vi "PosStrikerAnguloAttackerV2.vi"(9 "atacando contra":bool, 10 "IA State":T1={"our_robots"=[], "enemy_robots"=[], "balls"=[], "geometry"={"line_width"=0, "field_length"=0, "field_width"=0, "boundary_width"=0, "referee_width"=0, "goal_width"=0, "goal_depth"=0, "goal_wall_width"=0, "center_circle_radius"=0, "defense_radius"=0, "defense_stretch"=0, "free_kick_from_defense_dist"=0, "penalty_spot_from_field_line_dist"=0, "penalty_line_from_spot_dist"=0}, "IA Judge"={"stage"="", "command"="", "our_goalie_id"=0.0, "enemy_goalie_id"=0.0, "command enum"=enum."Halt", "Time"=enum."Azul"}, "Received Timestamp"=timestamp(0 s since 1904-01-01), "Events"={"Touch"=FALSE, "Ball out"=FALSE, "id touch"=0.0, "Ball out of \nVision"=FALSE, "Ball inside \nGoalie area"=FALSE, "Robot not responding"=FALSE, "Robots responding status"=[1.0, 1.0, 1.0, 1.0, 1.0, 1.0], "Enemy Ball \nPossession"=FALSE, "Pass State"=FALSE, "id end of pass"=0.0, "Kick"=FALSE, "Id ini Possession"=0.0, "Ball Possesion"=FALSE, "Id Possesion"=0.0, "Direct Kick"=FALSE}}) -> (0 "YdoAttacker 2":dbl, 1 "AttackerPositive?":bool, 2 "theta final":dbl, 3 "XdoAttacker 2":dbl)   [LabVIEW 2017]
uses:
  Core/AI Input.ctl
  Core/AI Robot.ctl
  Intel/Functions Enum.ctl
  Intel/AttackerStates.ctl
  Path Planning/RRT/PathDests.ctl
  Path Planning/RRT/PathDest.ctl
  Core/AI Ball.ctl
  Core/Field Size.ctl
  Core/AI Judge.ctl
  Intel/Command Enum.ctl
  Events/Events.ctl
panel:
  in  "valor de theta 3":dbl
  in  "tamanho do intervalo 3":dbl
  in  "inicio do intervalo 3":dbl
  in  "fim do intervalo 3":dbl
  in  "Contador 4":dbl
  in  "Array 3":dbl[](array[numeric])=[0.0, 0.0, 0.0, 0.0, 0.0, 0.0]
  in  "valor de theta 2":dbl
  in  "tamanho do intervalo 2":dbl
  in  "inicio do intervalo 2":dbl
  in  "fim do intervalo 2":dbl
  in  "Contador 3":dbl
  in  "Array 2":dbl[](array[numeric])=[0.0, 0.0, 0.0, 0.0, 0.0, 0.0]
  in  "XdoAttacker":dbl
  in  "YdoAttacker":dbl
  in  "RobôsParaAnalisar":dbl[][](array[numeric])=[[99999.0, 99999.0], [99999.0, 99999.0], [99999.0, 99999.0], [99999.0, 99999.0], [99999.0, 99999.0], [99999.0, 99999.0], [99999.0, 99999.0]]
  in  "Contador":dbl
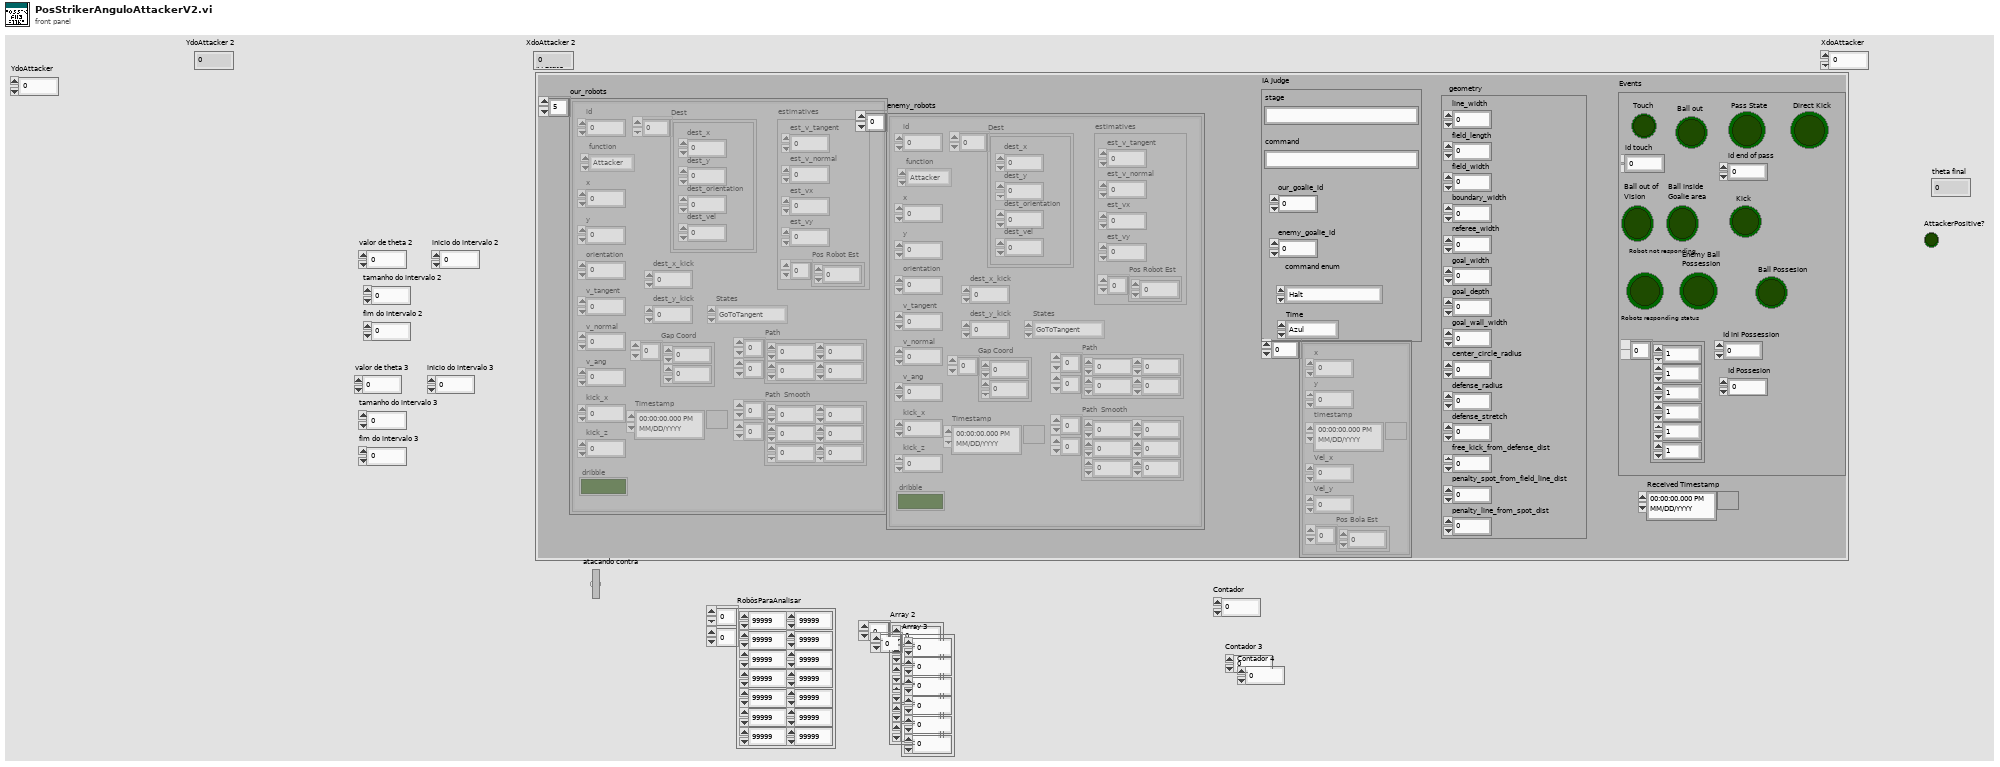
[diagram p1: front panel]
types:
  T1 = typedef "AI Input.ctl" = cluster{"our_robots":T2[], "enemy_robots":T2[], "balls":T7[], "geometry":T8, "IA Judge":T9, "Received Timestamp":timestamp, "Events":T11}
  T2 = typedef "AI Robot.ctl" = cluster{"id":u32, "function":T3, "x":dbl, "y":dbl, "orientation":dbl, "v_tangent":dbl, "v_normal":dbl, "v_ang":dbl, "kick_x":dbl, "kick_z":dbl, "dribble":bool, "Timestamp":timestamp, "estimatives":cluster{"est_v_tangent":dbl, "est_v_normal":dbl, "est_vx":dbl, "est_vy":dbl, "Pos Robot Est":dbl[]}, "dest_x_kick":dbl, "dest_y_kick":dbl, "Gap Coord":dbl[], "States":T4, "Path ":dbl[][], "Path  Smooth":dbl[][], "Dest":T5}
  T3 = typedef "Functions Enum.ctl" = enum16{"Attacker", "Goalie", "Defender", "Striker", "Goto 0", "Dummy", "Kicker", "ZigZag 0", "ZigZag 1", "ZigZag 2", "ZigZag 3", "ZigZag 4", "ZigZag 5", "ZigZag 6", "ZigZag 7", "ZigZag 8", ""}
  T4 = typedef "AttackerStates.ctl" = enum16{"Pass", "GoToTangent", "BallGetting", "GoToKick", ""}
  T5 = typedef "PathDests.ctl" = T6[]
  T6 = typedef "PathDest.ctl" = cluster{"dest_x":dbl, "dest_y":dbl, "dest_orientation":dbl, "dest_vel":dbl}
  T7 = typedef "AI Ball.ctl" = cluster{"x":dbl, "y":dbl, "timestamp":timestamp, "Vel_x":dbl, "Vel_y":dbl, "Pos Bola Est":dbl[]}
  T8 = typedef "Field Size.ctl" = cluster{"line_width":u32, "field_length":u32, "field_width":u32, "boundary_width":u32, "referee_width":u32, "goal_width":u32, "goal_depth":u32, "goal_wall_width":u32, "center_circle_radius":u32, "defense_radius":u32, "defense_stretch":u32, "free_kick_from_defense_dist":u32, "penalty_spot_from_field_line_dist":u32, "penalty_line_from_spot_dist":u32}
  T9 = typedef "AI Judge.ctl" = cluster{"stage":string, "command":string, "our_goalie_id":dbl, "enemy_goalie_id":dbl, "command enum":T10, "Time":enum16{"Azul", "Amarelo"}}
  T10 = typedef "Command Enum.ctl" = enum16{"Halt", "Stop", "Force Start", "PKA Normal Start", "Prepare Kickoff Ally", "PKE Normal Start", "Prepare Kickoff Enemy", "Prepare Penalty Ally", "PPA Normal Start", "Prepare Penalty Enemy", "PPE Normal Start", "Direct Free Enemy", "Direct Free Ally", "Indirect Free Enemy", "Indirect Free Ally", "Timeout Enemy", "Timeout Ally", "Goal Enemy", "Goal Ally", "Ball Placement Enemy", "Ball Placement Ally", "Normal Half Time", "Extra Time Break", "Extra Half Time", "None", "Post Game"}
  T11 = typedef "Events.ctl" = cluster{"Touch":bool, "Ball out":bool, "id touch":dbl, "Ball out of \nVision":bool, "Ball inside \nGoalie area":bool, "Robot not responding":bool, "Robots responding status":dbl[], "Enemy Ball \nPossession":bool, "Pass State":bool, "id end of pass":dbl, "Kick":bool, "Id ini Possession":dbl, "Ball Possesion":bool, "Id Possesion":dbl, "Direct Kick":bool}
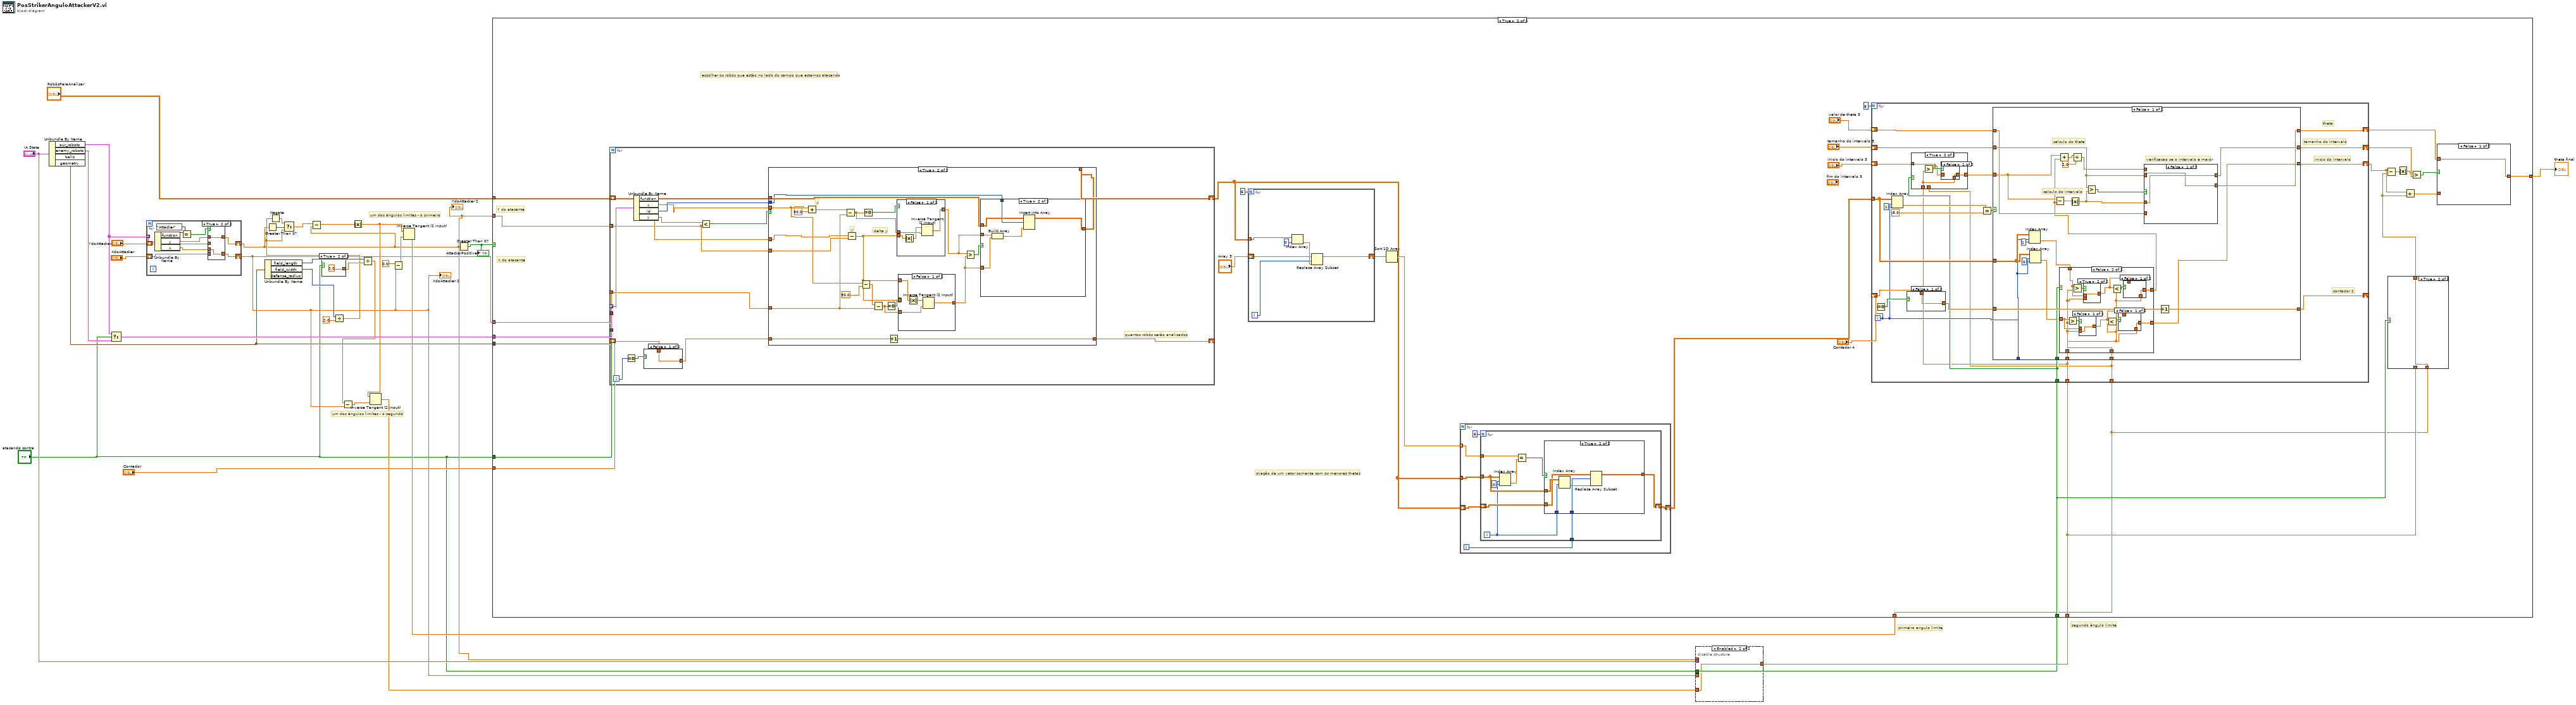
[diagram p0: block diagram]
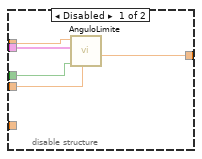
[diagram p2: hidden frame]
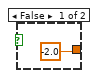
[diagram p3: hidden frame]
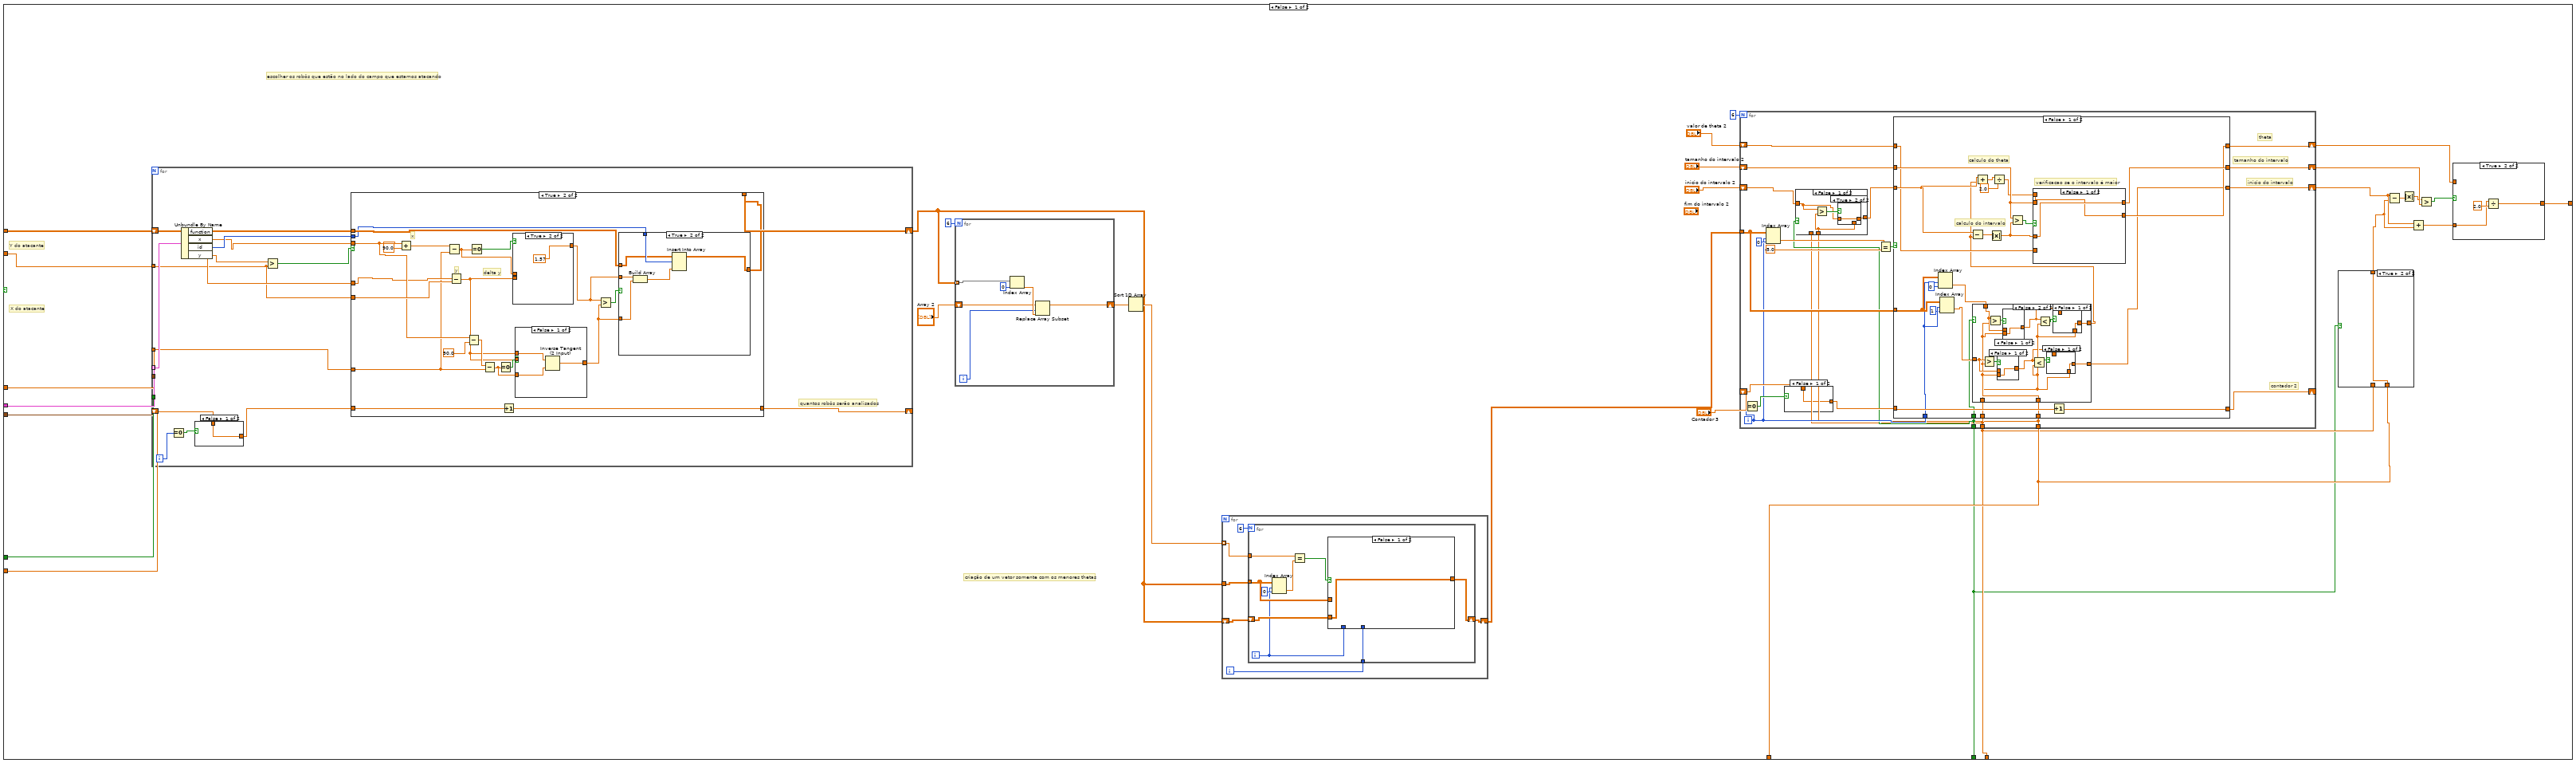
[diagram p4: hidden frame]
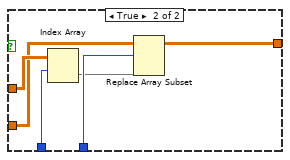
[diagram p7: hidden frame]
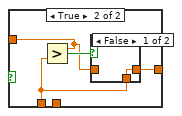
[diagram p9: hidden frame]
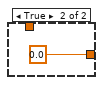
[diagram p11: hidden frame]
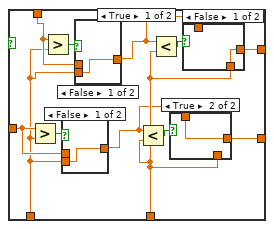
[diagram p12: hidden frame]
diagram:
  # "um dos ângulos limites - o segundo"
  # "primeiro angulo limite"
  # "segundo ãngulo limite"
  # "um dos ângulos limites - o primeiro"
  n1 = Unbundle By Name("IA State") -> ("our_robots"=w26:T2[], "enemy_robots"=w31:T2[], "geometry"=w18:T8)  [unwired: 1 out]
  n2 = Select(t=w26, s="atacando contra", f=w31) -> (s? t:f=w30:T2[])
  n3 = for {
    tunnel: w26 -> [w41] mode=indexing
    shift-right: [w36] -> w12
    shift-left: "YdoAttacker" -> [w35]
    shift-right: [w32] -> w2
    shift-left: "XdoAttacker" -> [w33]
    n4 = Unbundle By Name(w41) -> ("function"=w40:T3, "y"=w37:dbl, "x"=w34:dbl)
    n5 = Equal?(x=w40, y=Functions_Enum."Attacker") -> (x = y?=w38:bool)
    n6 = case shown="True" w38 {
      tunnel: w37 -> [_ w45]
      tunnel: [w43 w45] -> w36
      tunnel: w35 -> [w43 _]
      tunnel: w34 -> [_ w44]
      tunnel: w33 -> [w42 _]
      tunnel: [w42 w44] -> w32
      frame False {
      }
      frame True {
      }
    }
  }
  "YdoAttacker 2" <- w12
  "XdoAttacker 2" <- w2
  n7 = Unbundle By Name(w18) -> ("field_length"=w22:u32, "field_width"=w16:u32)  [unwired: 1 out]
  n8 = Greater Than 0?(x=w12) -> (x > 0?=w21:bool)
  n9 = case shown="True" "atacando contra" {
    tunnel: [-2.0 ("y") 2.0 ("y")] -> w19
    frame False {
    }
    frame True {
    }
  }
  n10 = Divide(x=w16, y=2.0) -> (x/y=w15:dbl)
  n11 = Negate(x=w15) -> (-x=w20:dbl)
  n12 = Select(t=w20, s=w21, f=w15) -> (s? t:f=w11:dbl)
  n13 = Subtract(x=w11, y=w12) -> (x-y=w9:dbl)
  n14 = Absolute Value(x=w9) -> (abs(x)=w4:dbl)
  n15 = Divide(x=w22, y=w19) -> (x/y=w6:dbl)
  n16 = Subtract(x=w6, y=w2) -> (x-y=w5:dbl)
  n17 = Inverse Tangent (2 Input)(1:w5, 2:w4) -> (0:w3:dbl)
  n18 = Subtract(x=0.0, y=w2) -> (x-y=w10:dbl)
  n19 = Inverse Tangent (2 Input)(1:w10, 2:w4) -> (0:w14:dbl)
  n20 = Greater Than 0?(x=w12) -> (x > 0?=w23:bool)
  "AttackerPositive?" <- w23
  n21 = disable-structure shown="Enabled" {
    disable-tunnel: [w48 w54] -> w13
    disable-tunnel: w12 -> [w53 _]
    disable-tunnel: "IA State" -> [w52 _]
    disable-tunnel: "atacando contra" -> [w51 _]
    disable-tunnel: w2 -> [w50 _]
    disable-tunnel: w3 -> [w49 w54]
    frame Disabled {
      n22 = call "AnguloLimite.vi"("XdoAttacker"=w50, "atacando contra"=w51, "IA State"=w52, "YdoAttacker"=w53) -> ("Angulo Limite"=w48:dbl)  [unwired: 7 in]
    }
    frame Enabled {
    }
  }
  n23 = case shown="True" w23 {
    tunnel: w30 -> [w84 w317]
    tunnel: "atacando contra" -> [w83 w316]
    tunnel: "Contador" -> [w82 w315]
    tunnel: "RobôsParaAnalisar" -> [w81 w314]
    tunnel: w18 -> [w80 w313]
    tunnel: [w66 w299] -> w27
    tunnel: w12 -> [w60 w293]
    tunnel: w2 -> [w59 w292]
    tunnel: w14 -> [w57 w288]
    tunnel: "atacando contra" -> [w55 w291]
    tunnel: w13 -> [w56 w290]
    frame False {
      # "X do atacante"
      # "Y do atacante"
      # "criação de um vetor somente com os menores thetas"
      # "escolher os robôs que estão no lado do campo que estamos atacando"
      n24 = for {
        tunnel: w84 -> [w238] mode=indexing
        tunnel: w83 -> [_]
        shift-right: [w230] -> w70
        shift-left: w81 -> [w237]
        shift-right: [w231] -> _
        shift-left: w82 -> [w233]
        tunnel: w80 -> [_]
        tunnel: w60 -> [w226]
        tunnel: w59 -> [w225]
        i -> [w234]
        # "quantos robôs serão analisados"
        n25 = Equal To 0?(x=w234) -> (x = 0?=w235:bool)
        n26 = Unbundle By Name(w238) -> ("x"=w229:dbl, "id"=w236:u32, "y"=w228:dbl)  [unwired: 1 out]
        n27 = case shown="False" w235 {
          tunnel: w233 -> [w239 _]
          tunnel: [w239 0.0] -> w232
          frame False {
          }
          frame True {
          }
        }
        n28 = Greater?(x=w228, y=w226) -> (0:w227:bool)
        n29 = case shown="True" w227 {
          tunnel: w237 -> [w245 w265]
          tunnel: w236 -> [w244 w264]
          tunnel: w229 -> [_ w255]
          tunnel: w228 -> [_ w254]
          tunnel: w232 -> [w246 w266]
          tunnel: [w246 w267] -> w231
          tunnel: [w241 w263] -> w230
          tunnel: w226 -> [_ w256]
          tunnel: w225 -> [_ w252]
          frame False {
            w243 = -5.0 ("element")
            n30 = Build Array(w243, w243) -> (w242:dbl[])
            n31 = Insert Into Array(array=w245, index (row)=w244, new element=w242) -> (w241:dbl[][])  [unwired: 1 in]
          }
          frame True {
            # "delta y"
            # "y"
            # "x"
            n32 = Add(x=w255, y=90.0) -> (x+y=w253:dbl)
            n33 = Subtract(x=w253, y=w252) -> (x-y=w250:dbl)
            n34 = Subtract(x=w254, y=w256) -> (x-y=w247:dbl)
            n35 = Subtract(x=w255, y=90.0) -> (x-y=w260:dbl)
            n36 = Equal To 0?(x=w250) -> (x = 0?=w251:bool)
            n37 = Subtract(x=w260, y=w252) -> (x-y=w248:dbl)
            n38 = Equal To 0?(x=w248) -> (x = 0?=w249:bool)
            n39 = Increment(x=w266) -> (x+1=w267:dbl)
            n40 = case shown="True" w251 {
              tunnel: [w285 1.57] -> w258
              tunnel: w247 -> [w286 _]
              tunnel: w250 -> [w284 _]
              frame False {
                n41 = Inverse Tangent (2 Input)(1:w284, 2:w286) -> (0:w285:dbl)
              }
              frame True {
              }
            }
            n42 = case shown="False" w249 {
              tunnel: [w270 1.57] -> w257
              tunnel: w247 -> [_ _]
              tunnel: w248 -> [w269 _]
              tunnel: w247 -> [w268 _]
              frame False {
                n43 = Inverse Tangent (2 Input)(1:w269, 2:w268) -> (0:w270:dbl)
              }
              frame True {
              }
            }
            n44 = Greater?(x=w258, y=w257) -> (0:w259:bool)
            n45 = case shown="True" w259 {
              tunnel: w265 -> [w274 w280]
              tunnel: w264 -> [w276 w283]
              tunnel: w258 -> [w273 w281]
              tunnel: w257 -> [w275 w279]
              tunnel: [w272 w278] -> w263
              frame False {
                n46 = Build Array(w275, w273) -> (w277:dbl[])
                n47 = Insert Into Array(array=w274, index (row)=w276, new element=w277) -> (w272:dbl[][])  [unwired: 1 in]
              }
              frame True {
                n48 = Build Array(w281, w279) -> (w282:dbl[])
                n49 = Insert Into Array(array=w280, index (row)=w283, new element=w282) -> (w278:dbl[][])  [unwired: 1 in]
              }
            }
          }
        }
      }
      n50 = for {
        N: 6 -> [_]
        tunnel: w70 -> [w118] mode=indexing
        shift-right: [w113] -> w72
        shift-left: "Array 2" -> [w114]
        i -> [w115]
        n51 = Index Array(array=w118, index=0) -> (element=w116:dbl)
        n52 = Replace Array Subset(array=w114, new element=w116, index=w115) -> (w113:dbl[])
      }
      n53 = Sort 1D Array(array=w72) -> (sorted array=w71:dbl[])
      n54 = for {
        tunnel: w71 -> [w93] mode=indexing
        tunnel: w70 -> [w95]
        shift-right: [w91] -> w69
        shift-left: w70 -> [w94]
        i -> [w92]
        n55 = for {
          N: 6 -> [_]
          tunnel: w95 -> [w101]
          shift-right: [w97] -> w91
          shift-left: w94 -> [w100]
          tunnel: w93 -> [w103]
          tunnel: w92 -> [w98]
          i -> [w99]
          n56 = Index Array(array=w101, index (row)=w99, index (col)=0 ("disabled index (col)")) -> (element=w104:dbl)
          n57 = Equal?(x=w103, y=w104) -> (x = y?=w102:bool)
          n58 = case shown="False" w102 {
            tunnel: w101 -> [_ w112]
            tunnel: w100 -> [w106 w108]
            tunnel: w99 -> [_ w111]
            tunnel: w98 -> [_ w110]
            tunnel: [w106 w107] -> w97
            frame False {
            }
            frame True {
              n59 = Index Array(array=w112, index (row)=w111) -> (element=w109:dbl[])  [unwired: 1 in]
              n60 = Replace Array Subset(array=w108, new element=w109, index (row)=w110) -> (w107:dbl[][])  [unwired: 1 in]
            }
          }
        }
      }
      n61 = for {
        N: 6 -> [_]
        tunnel: w69 -> [w125]
        shift-right: [w133] -> w65
        shift-left: "valor de theta 2" -> [w134]
        shift-right: [w131] -> w68
        shift-left: "tamanho do intervalo 2" -> [w132]
        shift-right: [w130] -> w62
        shift-left: "inicio do intervalo 2" -> [w122]
        shift-right: [w126] -> _
        shift-left: "Contador 3" -> [w128]
        tunnel: w56 -> [w120]
        tunnel: w57 -> [w119]
        tunnel: w55 -> [w123]
        i -> [w124]
        # "contador 2"
        # "inicio do intervalo"
        # "tamanho do intervalo"
        # "theta"
        n62 = Equal To 0?(x=w124) -> (x = 0?=w129:bool)
        n63 = Index Array(array=w125, index (row)=w124, index (col)=0 ("disabled index (col)")) -> (element=w136:dbl)
        n64 = case shown="False" w129 {
          tunnel: w128 -> [w151 _]
          tunnel: [w151 0.0] -> w127
          frame False {
          }
          frame True {
          }
        }
        n65 = case shown="False" w123 {
          tunnel: w120 -> [_ w145]
          tunnel: w122 -> [w141 w146]
          tunnel: [w139 w147] -> w121
          tunnel: w119 -> [w140 _]
          frame False {
            n66 = Greater?(x=w141, y=w140) -> (0:w142:bool)
            n67 = case shown="True" w142 {
              tunnel: [w143 w144] -> w139
              tunnel: w141 -> [_ w144]
              tunnel: w140 -> [w143 _]
              frame False {
              }
              frame True {
              }
            }
          }
          frame True {
            n68 = Greater?(x=w146, y=w145) -> (0:w148:bool)
            n69 = case shown="False" w148 {
              tunnel: [w149 w150] -> w147
              tunnel: w146 -> [_ w150]
              tunnel: w145 -> [w149 _]
              frame False {
              }
              frame True {
              }
            }
          }
        }
        n70 = Equal?(x=w136, y=-5.0) -> (x = y?=w137:bool)
        n71 = case shown="False" w137 {
          tunnel: w134 -> [w160 w224]
          tunnel: [w161 w224] -> w133
          tunnel: w132 -> [w165 w223]
          tunnel: [w164 w223] -> w131
          tunnel: w121 -> [w176 w222]
          tunnel: [w158 w222] -> w130
          tunnel: w127 -> [w174 w221]
          tunnel: [w175 w221] -> w126
          tunnel: w125 -> [w173 _]
          tunnel: w124 -> [w172 _]
          tunnel: w120 -> [w155 _]
          tunnel: w119 -> [w154 _]
          tunnel: w123 -> [w153 _]
          frame False {
            # "calculo do theta"
            # "calculo do intervalo"
            # "verificacao se o intervalo é maior"
            n72 = Index Array(array=w173, index (row)=w172, index (col)=0 ("disabled index (col)")) -> (element=w157:dbl)
            n73 = Index Array(array=w173, index (row)=w172, index (col)=1 ("disabled index (col)")) -> (element=w159:dbl)
            n74 = case shown="False" w153 {
              tunnel: w155 -> [w180 w198]
              tunnel: w157 -> [w187 w207]
              tunnel: w154 -> [w179 w199]
              tunnel: [w185 w205] -> w156
              tunnel: w159 -> [w181 w201]
              tunnel: [w178 w200] -> w158
              frame True {
                n75 = Greater?(x=w181, y=w180) -> (0:w183:bool)
                n76 = Greater?(x=w187, y=w180) -> (0:w188:bool)
                n77 = case shown="False" w183 {
                  tunnel: [w191 w192] -> w177
                  tunnel: w181 -> [_ w192]
                  tunnel: w180 -> [w191 _]
                  frame False {
                  }
                  frame True {
                  }
                }
                n78 = case shown="False" w188 {
                  tunnel: [w195 w196] -> w184
                  tunnel: w187 -> [_ w196]
                  tunnel: w180 -> [w195 _]
                  frame False {
                  }
                  frame True {
                  }
                }
                n79 = Less?(x=w177, y=w179) -> (x < y?=w182:bool)
                n80 = Less?(x=w184, y=w179) -> (x < y?=w186:bool)
                n81 = case shown="True" w182 {
                  tunnel: [w189 w190] -> w178
                  tunnel: w177 -> [_ w190]
                  tunnel: w179 -> [w189 _]
                  frame False {
                  }
                  frame True {
                  }
                }
                n82 = case shown="False" w186 {
                  tunnel: [w193 w194] -> w185
                  tunnel: w184 -> [_ w194]
                  tunnel: w179 -> [w193 _]
                  frame False {
                  }
                  frame True {
                  }
                }
              }
              frame False {
                n83 = Greater?(x=w201, y=w199) -> (0:w203:bool)
                n84 = Greater?(x=w207, y=w199) -> (0:w208:bool)
                n85 = case shown="False" w203 {
                  tunnel: [w211 w212] -> w197
                  tunnel: w201 -> [_ w212]
                  tunnel: w199 -> [w211 _]
                  frame False {
                  }
                  frame True {
                  }
                }
                n86 = case shown="False" w208 {
                  tunnel: [w215 w216] -> w204
                  tunnel: w207 -> [_ w216]
                  tunnel: w199 -> [w215 _]
                  frame False {
                  }
                  frame True {
                  }
                }
                n87 = Less?(x=w197, y=w198) -> (x < y?=w202:bool)
                n88 = Less?(x=w204, y=w198) -> (x < y?=w206:bool)
                n89 = case shown="False" w202 {
                  tunnel: [w209 w210] -> w200
                  tunnel: w197 -> [_ w210]
                  tunnel: w198 -> [w209 _]
                  frame False {
                  }
                  frame True {
                  }
                }
                n90 = case shown="False" w206 {
                  tunnel: [w213 w214] -> w205
                  tunnel: w204 -> [_ w214]
                  tunnel: w198 -> [w213 _]
                  frame False {
                  }
                  frame True {
                  }
                }
              }
            }
            n91 = Subtract(x=w176, y=w156) -> (x-y=w169:dbl)
            n92 = Add(x=w176, y=w156) -> (x+y=w168:dbl)
            n93 = Absolute Value(x=w169) -> (abs(x)=w163:dbl)
            n94 = Divide(x=w168, y=2.0) -> (x/y=w162:dbl)
            n95 = Greater?(x=w165, y=w163) -> (0:w166:bool)
            n96 = case shown="False" w166 {
              tunnel: w165 -> [_ w220]
              tunnel: [w218 w220] -> w164
              tunnel: w163 -> [w218 _]
              tunnel: w160 -> [_ w219]
              tunnel: w162 -> [w217 _]
              tunnel: [w217 w219] -> w161
              frame False {
              }
              frame True {
              }
            }
            n97 = Increment(x=w174) -> (x+1=w175:dbl)
          }
          frame True {
          }
        }
      }
      n98 = case shown="True" w55 {
        tunnel: w56 -> [w85 _]
        tunnel: [w85 w86] -> w58
        tunnel: w57 -> [_ w86]
        frame False {
        }
        frame True {
        }
      }
      n99 = Subtract(x=w62, y=w58) -> (x-y=w64:dbl)
      n100 = Absolute Value(x=w64) -> (abs(x)=w63:dbl)
      n101 = Add(x=w62, y=w58) -> (x+y=w61:dbl)
      n102 = Greater?(x=w63, y=w68) -> (0:w67:bool)
      n103 = case shown="True" w67 {
        tunnel: [w87 w89] -> w66
        tunnel: w65 -> [w87 _]
        tunnel: w61 -> [_ w88]
        frame False {
        }
        frame True {
          n104 = Divide(x=w88, y=2.0) -> (x/y=w89:dbl)
        }
      }
    }
    frame True {
      # "X do atacante"
      # "Y do atacante"
      # "criação de um vetor somente com os menores thetas"
      # "escolher os robôs que estão no lado do campo que estamos atacando"
      n105 = for {
        tunnel: w317 -> [w471] mode=indexing
        tunnel: w316 -> [_]
        shift-right: [w463] -> w303
        shift-left: w314 -> [w470]
        shift-right: [w464] -> _
        shift-left: w315 -> [w466]
        tunnel: w313 -> [_]
        tunnel: w293 -> [w459]
        tunnel: w292 -> [w458]
        i -> [w467]
        # "quantos robôs serão analisados"
        n106 = Equal To 0?(x=w467) -> (x = 0?=w468:bool)
        n107 = Unbundle By Name(w471) -> ("x"=w462:dbl, "id"=w469:u32, "y"=w461:dbl)  [unwired: 1 out]
        n108 = case shown="False" w468 {
          tunnel: w466 -> [w472 _]
          tunnel: [w472 0.0] -> w465
          frame False {
          }
          frame True {
          }
        }
        n109 = Less?(x=w461, y=w459) -> (x < y?=w460:bool)
        n110 = case shown="True" w460 {
          tunnel: w470 -> [w478 w498]
          tunnel: w469 -> [w477 w497]
          tunnel: w462 -> [_ w488]
          tunnel: w461 -> [_ w487]
          tunnel: w465 -> [w479 w499]
          tunnel: [w479 w500] -> w464
          tunnel: [w474 w496] -> w463
          tunnel: w459 -> [_ w489]
          tunnel: w458 -> [_ w485]
          frame False {
            w476 = -5.0 ("element")
            n111 = Build Array(w476, w476) -> (w475:dbl[])
            n112 = Insert Into Array(array=w478, index (row)=w477, new element=w475) -> (w474:dbl[][])  [unwired: 1 in]
          }
          frame True {
            # "delta y"
            # "y"
            # "x"
            n113 = Add(x=w488, y=90.0) -> (x+y=w486:dbl)
            n114 = Subtract(x=w486, y=w485) -> (x-y=w483:dbl)
            n115 = Subtract(x=w487, y=w489) -> (x-y=w480:dbl)
            n116 = Subtract(x=w488, y=90.0) -> (x-y=w493:dbl)
            n117 = Equal To 0?(x=w483) -> (x = 0?=w484:bool)
            n118 = Subtract(x=w493, y=w485) -> (x-y=w481:dbl)
            n119 = Equal To 0?(x=w481) -> (x = 0?=w482:bool)
            n120 = Increment(x=w499) -> (x+1=w500:dbl)
            n121 = case shown="False" w484 {
              tunnel: [w521 1.57] -> w491
              tunnel: w480 -> [w519 _]
              tunnel: w483 -> [w520 _]
              frame False {
                n122 = Absolute Value(x=w519) -> (abs(x)=w518:dbl)
                n123 = Inverse Tangent (2 Input)(1:w520, 2:w518) -> (0:w521:dbl)
              }
              frame True {
              }
            }
            n124 = case shown="False" w482 {
              tunnel: [w504 1.57] -> w490
              tunnel: w480 -> [_ _]
              tunnel: w481 -> [w503 _]
              tunnel: w480 -> [w501 _]
              frame False {
                n125 = Absolute Value(x=w501) -> (abs(x)=w502:dbl)
                n126 = Inverse Tangent (2 Input)(1:w503, 2:w502) -> (0:w504:dbl)
              }
              frame True {
              }
            }
            n127 = Greater?(x=w491, y=w490) -> (0:w492:bool)
            n128 = case shown="True" w492 {
              tunnel: w498 -> [w508 w514]
              tunnel: w497 -> [w510 w517]
              tunnel: w491 -> [w507 w515]
              tunnel: w490 -> [w509 w513]
              tunnel: [w506 w512] -> w496
              frame False {
                n129 = Build Array(w509, w507) -> (w511:dbl[])
                n130 = Insert Into Array(array=w508, index (row)=w510, new element=w511) -> (w506:dbl[][])  [unwired: 1 in]
              }
              frame True {
                n131 = Build Array(w515, w513) -> (w516:dbl[])
                n132 = Insert Into Array(array=w514, index (row)=w517, new element=w516) -> (w512:dbl[][])  [unwired: 1 in]
              }
            }
          }
        }
      }
      n133 = for {
        N: 6 -> [_]
        tunnel: w303 -> [w351] mode=indexing
        shift-right: [w346] -> w305
        shift-left: "Array 3" -> [w347]
        i -> [w348]
        n134 = Index Array(array=w351, index=0) -> (element=w349:dbl)
        n135 = Replace Array Subset(array=w347, new element=w349, index=w348) -> (w346:dbl[])
      }
      n136 = Sort 1D Array(array=w305) -> (sorted array=w304:dbl[])
      n137 = for {
        tunnel: w304 -> [w326] mode=indexing
        tunnel: w303 -> [w328]
        shift-right: [w324] -> w302
        shift-left: w303 -> [w327]
        i -> [w325]
        n138 = for {
          N: 6 -> [_]
          tunnel: w328 -> [w334]
          shift-right: [w330] -> w324
          shift-left: w327 -> [w333]
          tunnel: w326 -> [w336]
          tunnel: w325 -> [w331]
          i -> [w332]
          n139 = Index Array(array=w334, index (row)=w332, index (col)=0 ("disabled index (col)")) -> (element=w337:dbl)
          n140 = Equal?(x=w336, y=w337) -> (x = y?=w335:bool)
          n141 = case shown="True" w335 {
            tunnel: w334 -> [_ w345]
            tunnel: w333 -> [w339 w341]
            tunnel: w332 -> [_ w344]
            tunnel: w331 -> [_ w343]
            tunnel: [w339 w340] -> w330
            frame False {
            }
            frame True {
              n142 = Index Array(array=w345, index (row)=w344) -> (element=w342:dbl[])  [unwired: 1 in]
              n143 = Replace Array Subset(array=w341, new element=w342, index (row)=w343) -> (w340:dbl[][])  [unwired: 1 in]
            }
          }
        }
      }
      n144 = for {
        N: 6 -> [_]
        tunnel: w302 -> [w358]
        shift-right: [w366] -> w298
        shift-left: "valor de theta 3" -> [w367]
        shift-right: [w364] -> w301
        shift-left: "tamanho do intervalo 3" -> [w365]
        shift-right: [w363] -> w295
        shift-left: "inicio do intervalo 3" -> [w354]
        shift-right: [w359] -> _
        shift-left: "Contador 4" -> [w361]
        tunnel: w291 -> [w356]
        tunnel: w290 -> [w355]
        tunnel: w288 -> [w352]
        i -> [w357]
        # "contador 2"
        # "inicio do intervalo"
        # "tamanho do intervalo"
        # "theta"
        n145 = Equal To 0?(x=w357) -> (x = 0?=w362:bool)
        n146 = Index Array(array=w358, index (row)=w357, index (col)=1 ("disabled index (col)")) -> (element=w369:dbl)
        n147 = case shown="False" w362 {
          tunnel: w361 -> [w384 _]
          tunnel: [w384 0.0] -> w360
          frame False {
          }
          frame True {
          }
        }
        n148 = case shown="True" w356 {
          tunnel: w355 -> [_ w378]
          tunnel: w354 -> [w374 w379]
          tunnel: [w372 w380] -> w353
          tunnel: w352 -> [w373 _]
          frame False {
            n149 = Greater?(x=w374, y=w373) -> (0:w375:bool)
            n150 = case shown="True" w375 {
              tunnel: [w376 w377] -> w372
              tunnel: w374 -> [_ w377]
              tunnel: w373 -> [w376 _]
              frame False {
              }
              frame True {
              }
            }
          }
          frame True {
            n151 = Greater?(x=w379, y=w378) -> (0:w381:bool)
            n152 = case shown="False" w381 {
              tunnel: [w382 w383] -> w380
              tunnel: w379 -> [_ w383]
              tunnel: w378 -> [w382 _]
              frame False {
              }
              frame True {
              }
            }
          }
        }
        n153 = Equal?(x=w369, y=-5.0) -> (x = y?=w370:bool)
        n154 = case shown="False" w370 {
          tunnel: w367 -> [w394 w457]
          tunnel: [w395 w457] -> w366
          tunnel: w365 -> [w399 w456]
          tunnel: [w398 w456] -> w364
          tunnel: [w388 w454] -> w363
          tunnel: w360 -> [w408 w455]
          tunnel: [w409 w455] -> w359
          tunnel: w358 -> [w407 _]
          tunnel: w357 -> [w406 _]
          tunnel: w356 -> [w393 _]
          tunnel: w355 -> [w392 _]
          tunnel: w352 -> [w391 _]
          tunnel: w353 -> [w387 w454]
          frame False {
            # "calculo do theta"
            # "calculo do intervalo"
            # "verificacao se o intervalo é maior"
            n155 = Index Array(array=w407, index (row)=w406, index (col)=1 ("disabled index (col)")) -> (element=w386:dbl)
            n156 = Index Array(array=w407, index (row)=w406, index (col)=0 ("disabled index (col)")) -> (element=w389:dbl)
            n157 = case shown="False" w393 {
              tunnel: w392 -> [w413 w431]
              tunnel: w386 -> [w420 w440]
              tunnel: w391 -> [w412 w432]
              tunnel: [w418 w438] -> w390
              tunnel: w389 -> [w414 w434]
              tunnel: [w411 w433] -> w388
              frame True {
                n158 = Greater?(x=w414, y=w413) -> (0:w416:bool)
                n159 = Greater?(x=w420, y=w413) -> (0:w421:bool)
                n160 = case shown="False" w416 {
                  tunnel: [w424 w425] -> w410
                  tunnel: w414 -> [_ w425]
                  tunnel: w413 -> [w424 _]
                  frame False {
                  }
                  frame True {
                  }
                }
                n161 = case shown="False" w421 {
                  tunnel: [w428 w429] -> w417
                  tunnel: w420 -> [_ w429]
                  tunnel: w413 -> [w428 _]
                  frame False {
                  }
                  frame True {
                  }
                }
                n162 = Less?(x=w410, y=w412) -> (x < y?=w415:bool)
                n163 = Less?(x=w417, y=w412) -> (x < y?=w419:bool)
                n164 = case shown="True" w415 {
                  tunnel: [w422 w423] -> w411
                  tunnel: w410 -> [_ w423]
                  tunnel: w412 -> [w422 _]
                  frame False {
                  }
                  frame True {
                  }
                }
                n165 = case shown="True" w419 {
                  tunnel: [w426 w427] -> w418
                  tunnel: w417 -> [_ w427]
                  tunnel: w412 -> [w426 _]
                  frame False {
                  }
                  frame True {
                  }
                }
              }
              frame False {
                n166 = Greater?(x=w434, y=w432) -> (0:w436:bool)
                n167 = Greater?(x=w440, y=w432) -> (0:w441:bool)
                n168 = case shown="False" w436 {
                  tunnel: [w444 w445] -> w430
                  tunnel: w434 -> [_ w445]
                  tunnel: w432 -> [w444 _]
                  frame False {
                  }
                  frame True {
                  }
                }
                n169 = case shown="True" w441 {
                  tunnel: [w448 w449] -> w437
                  tunnel: w440 -> [_ w449]
                  tunnel: w432 -> [w448 _]
                  frame False {
                  }
                  frame True {
                  }
                }
                n170 = Less?(x=w430, y=w431) -> (x < y?=w435:bool)
                n171 = Less?(x=w437, y=w431) -> (x < y?=w439:bool)
                n172 = case shown="False" w435 {
                  tunnel: [w442 w443] -> w433
                  tunnel: w430 -> [_ w443]
                  tunnel: w431 -> [w442 _]
                  frame False {
                  }
                  frame True {
                  }
                }
                n173 = case shown="False" w439 {
                  tunnel: [w446 w447] -> w438
                  tunnel: w437 -> [_ w447]
                  tunnel: w431 -> [w446 _]
                  frame False {
                  }
                  frame True {
                  }
                }
              }
            }
            n174 = Subtract(x=w387, y=w390) -> (x-y=w403:dbl)
            n175 = Add(x=w387, y=w390) -> (x+y=w402:dbl)
            n176 = Absolute Value(x=w403) -> (abs(x)=w397:dbl)
            n177 = Divide(x=w402, y=2.0) -> (x/y=w396:dbl)
            n178 = Greater?(x=w399, y=w397) -> (0:w400:bool)
            n179 = case shown="False" w400 {
              tunnel: w399 -> [_ w453]
              tunnel: [w451 w453] -> w398
              tunnel: w397 -> [w451 _]
              tunnel: w394 -> [_ w452]
              tunnel: w396 -> [w450 _]
              tunnel: [w450 w452] -> w395
              frame False {
              }
              frame True {
              }
            }
            n180 = Increment(x=w408) -> (x+1=w409:dbl)
          }
          frame True {
          }
        }
      }
      n181 = case shown="True" w291 {
        tunnel: w290 -> [w318 _]
        tunnel: [w318 w319] -> w289
        tunnel: w288 -> [_ w319]
        frame False {
        }
        frame True {
        }
      }
      n182 = Subtract(x=w295, y=w289) -> (x-y=w297:dbl)
      n183 = Absolute Value(x=w297) -> (abs(x)=w296:dbl)
      n184 = Add(x=w295, y=w289) -> (x+y=w294:dbl)
      n185 = Greater?(x=w296, y=w301) -> (0:w300:bool)
      n186 = case shown="False" w300 {
        tunnel: [w320 w322] -> w299
        tunnel: w298 -> [w320 _]
        tunnel: w294 -> [_ w321]
        frame False {
        }
        frame True {
          n187 = Divide(x=w321, y=2.0) -> (x/y=w322:dbl)
        }
      }
    }
  }
  "theta final" <- w27
